vi "SubVI_ProcessImage.vi"(0 "Image Path":path, 1 "Path to Python.exe":path=path "Python", 2 "Initial Guess":T1={"Center (pixels)"=-1.0, "Reflectivity"=0.0} {"Center (pixels)" format="%#_16g"}) -> (3 "Success":bool, 4 "Params Vector":dbl[](array[numeric]) format="%#_10f", 5 "Errors":dbl[](array[numeric]) format="%#_2g", 6 "Iterations":i32)   [LabVIEW 2016]
panel:
  out "error out":errorcluster
  out "Graph of Final Fit":cluster{dbl[], dbl[]}[](graph) caption="XY Graph"
  out "standard error":string
  out "return code":i32
  # "1. Imputs"
  # "2. Outputs"
  # "Center (px)"
  # "Reflectivity (ul)"
  # "Amplitude (px val^2)"
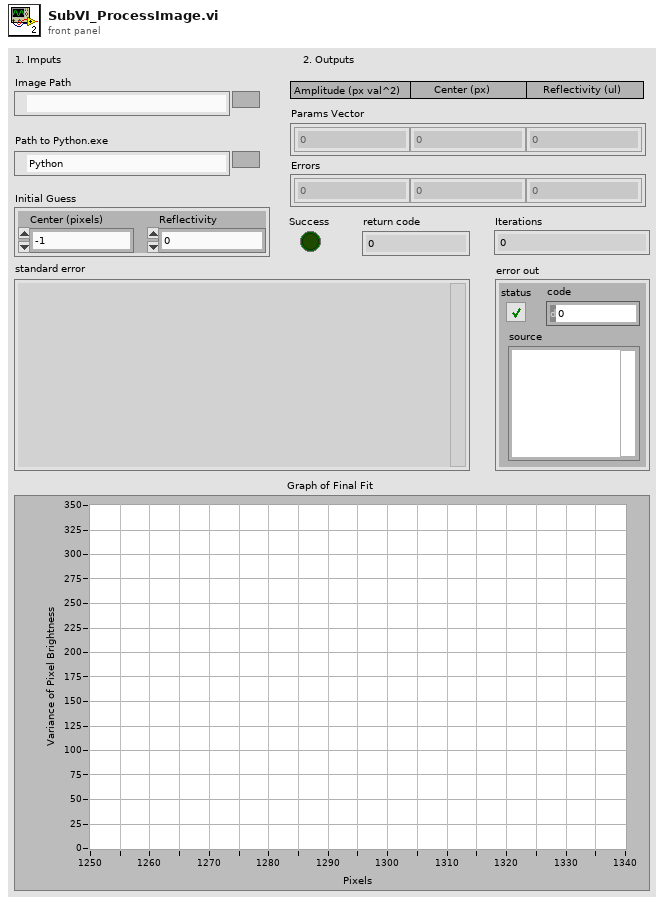
[diagram p1: front panel]
types:
  T1 = cluster{"Center (pixels)":dbl, "Reflectivity":dbl}
  T2 = cluster{"Image Path":path, "Initial Guess":cluster{"Center (pixels)":dbl, "Reflectivity":dbl}}
  T3 = cluster{dbl[], dbl[], i32, cluster{dbl[], dbl[], dbl[]}}
  T4 = enum8{"Enabled", "Disabled", "Disabled and Grayed Out"}
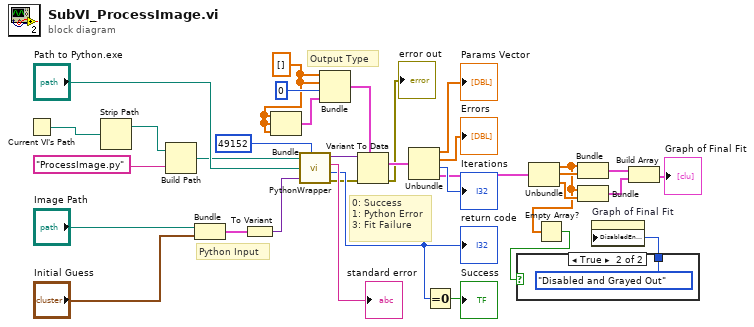
[diagram p0: block diagram]
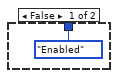
[diagram p2: hidden frame]
diagram:
  w12 = dbl[] []
  # "0: Success\n1: Python Error\n3: Fit Failure"
  # "Python Input"
  # "Output Type"
  n1 = Current VI's Path() -> (path=w33:path)
  n2 = Strip Path(path=w33) -> (stripped path=w20:path)  [unwired: 1 out]
  n3 = Build Path(base path=w20, name or relative path="ProcessImage.py") -> (appended path=w21:path)
  n4 = Bundle("Image Path"="Image Path", "Initial Guess"="Initial Guess") -> (w19:T2)  [unwired: 1 in]
  n5 = To Variant(anything=w19) -> (Variant=w30:variant)
  n6 = Bundle(w12, w12, w12) -> (w13:cluster{dbl[], dbl[], dbl[]})  [unwired: 1 in]
  n7 = call "PythonWrapper.vi"("file to run"=w21, "expected output size (4096)"=u32 49152, "Python.exe"="Path to Python.exe", "data in"=w30) -> ("data out"=w28:variant, "standard error"=→"standard error":string, "return code"=w17:i32, "error out"=w16:errorcluster)  [unwired: 1 in]
  "return code" <- w17
  n8 = Bundle(w12, w12, 0, w13) -> (w26:T3)  [unwired: 1 in]
  n9 = Variant To Data(error in=w16, type=w26, Variant=w28) -> (data=w25:T3, error out=→"error out":errorcluster)
  n10 = Unbundle(w25) -> (→"Params Vector":dbl[], →"Errors":dbl[], →"Iterations":i32, w11:cluster{dbl[], dbl[], dbl[]})
  n11 = Equal To 0?(x=w17) -> (x = 0?=→"Success":bool)
  n12 = Unbundle(w11) -> (w3:dbl[], w10:dbl[], w9:dbl[])
  n13 = Empty Array?(array=w3) -> (empty?=w2:bool)
  n14 = case shown="True" w2 {
    tunnel: [T4."Enabled" ("Disabled") T4."Disabled and Grayed Out" ("Disabled")] -> w4
    frame False {
    }
    frame True {
    }
  }
  n15 = Bundle(w3, w10) -> (w7:cluster{dbl[], dbl[]})  [unwired: 1 in]
  n16 = Bundle(w3, w9) -> (w6:cluster{dbl[], dbl[]})  [unwired: 1 in]
  n17 = property on="Graph of Final Fit" class="XYGraph (strict)"("DisabledEnum"=w4) -> ()  [unwired: 2 in, 2 out]
  n18 = Build Array(w7, w6) -> (→"Graph of Final Fit":cluster{dbl[], dbl[]}[])
